vi "GLOBALDriveTrain.vi"() -> ()   [LabVIEW 2011]
panel:
  in  "Servo Positions":T1={"Shifting"={"Right Servo High"=0.9, "Right Servo Low"=0.6, "Left Servo High"=0.0, "Left Servo Low"=0.7}, "Breaking"={"Coast Position"=0.05, "Break Position"=0.2}}
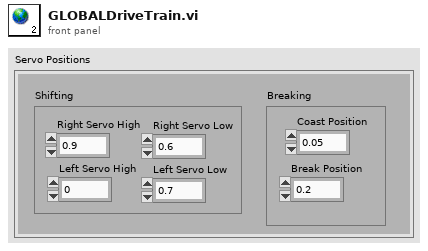
[diagram p1: front panel]
types:
  T1 = cluster{"Shifting":cluster{"Right Servo High":dbl, "Right Servo Low":dbl, "Left Servo High":dbl, "Left Servo Low":dbl}, "Breaking":cluster{"Coast Position":dbl, "Break Position":dbl}}
diagram:
